vi "Determine Where to Add.vi"(8 "error in (no error)":errorcluster, 11 "QControlWizard in":refnum<class "QControl Creation Wizard.lvclass">) -> (0 "error out":errorcluster, 3 "QControlWizard (dup)":refnum<class "QControl Creation Wizard.lvclass">)   [LabVIEW 2015, in "QControl Creation Wizard.lvclass"]
doc: "<b> </b> <b> </b>\n©2016 Q Software Innovations, LLC (QSI)\nwritten by Quentin Alldredge\nproduced in LabVIEW 2015\n\nsupport@qsoftwareinnovations.com\nwww.qsoftwareinnovations.com\n\nAll rights reserved.\n\nRedistribution and use in source and binary forms, with or without modification, are permitted provided that the following conditions are met:\n\n * Redistributions of source code must retain the above copyright notice, this list of conditions and the following disclaimer.\n * Redistributions in binary form must reproduce the above copyright notice, this list of conditions and the following disclaimer in the documentation and/or other materials provided with the distribution.\n * Neither the name of Q Software Innovations, LLC. nor the names of its contributors may be used to endorse or promote products derived from this software without specific prior written permission.\n\nTHIS SOFTWARE IS PROVIDED BY THE COPYRIGHT HOLDERS AND CONTRIBUTORS \"AS IS\" AND ANY EXPRESS OR IMPLIED WARRANTIES, INCLUDING, BUT NOT LIMITED TO, THE IMPLIED WARRANTIES OF MERCHANTABILITY AND FITNESS FOR A PARTICULAR PURPOSE ARE DISCLAIMED. IN NO EVENT SHALL THE COPYRIGHT OWNER OR CONTRIBUTORS BE LIABLE FOR ANY DIRECT, INDIRECT, INCIDENTAL, SPECIAL, EXEMPLARY, OR CONSEQUENTIAL DAMAGES (INCLUDING, BUT NOT LIMITED TO, PROCUREMENT OF SUBSTITUTE GOODS OR SERVICES; LOSS OF USE, DATA, OR PROFITS; OR BUSINESS INTERRUPTION) HOWEVER CAUSED AND ON ANY THEORY OF LIABILITY, WHETHER IN CONTRACT, STRICT LIABILITY, OR TORT (INCLUDING NEGLIGENCE OR OTHERWISE) ARISING IN ANY WAY OUT OF THE USE OF THIS SOFTWARE, EVEN IF ADVISED OF THE POSSIBILITY OF SUCH DAMAGE."
uses:
  QControl Creation Wizard.lvclass
  QControl Creation Wizard.lvclass/QControl Creation Wizard.ctl
  New QControl Info/New QControl Info.lvclass/New QControl Info.ctl
  New QControl Info/Write Add to Location.vi
  New QControl Info/Write ProjectItem Ref.vi
  New QControl Info/Write Target Ref.vi
  New QControl Info/Read App Refnum.vi
  New QControl Info/New QControl Info.lvclass
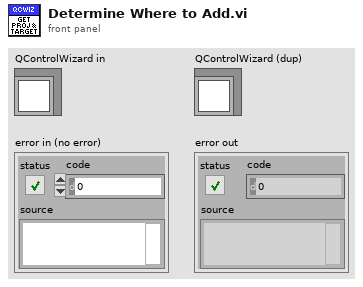
[diagram p1: front panel]
types:
  T1 = enum16{"Don't Add", "To Target", "To Project Item"}
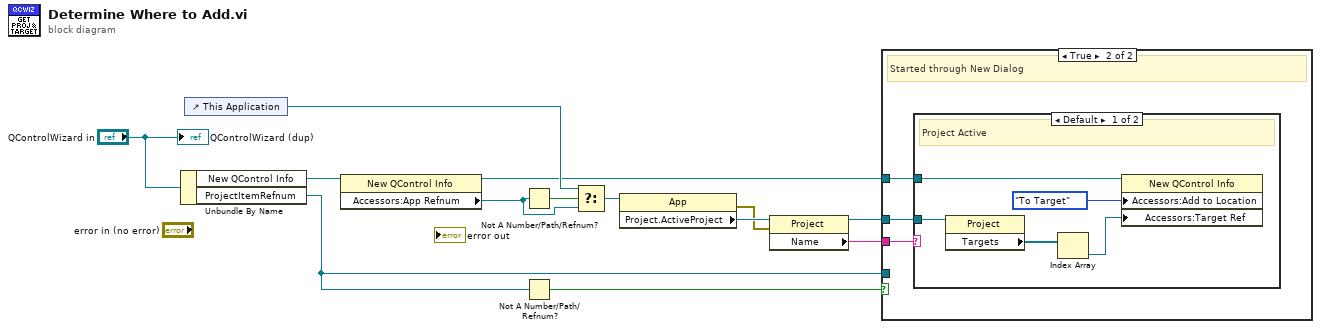
[diagram p0: block diagram]
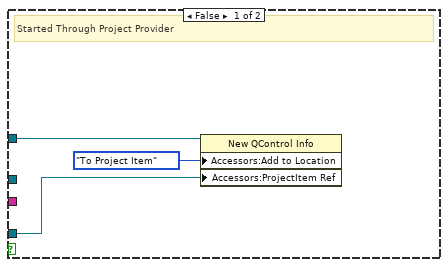
[diagram p2: hidden frame]
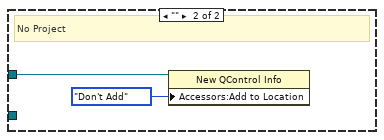
[diagram p3: hidden frame]
diagram:
  n1 = Unbundle By Name("QControlWizard in") -> ("New QControl Info"=w4:refnum<data-value>, "ProjectItemRefnum"=w5:refnum<vi>)
  n2 = control-ref of="This Application"() -> (w9:refnum<vi>)
  n3 = property class="New QControl Info"(reference=w4) -> (reference out=w2:refnum<data-value>, "Accessors:App Refnum"=w1:refnum<vi>)  [unwired: 1 in, 1 out]
  n4 = Not A Number/Path/Refnum?(number/path/refnum=w1) -> (NaN/Path/Refnum?=w11:bool)
  n5 = Not A Number/Path/Refnum?(number/path/refnum=w5) -> (NaN/Path/Refnum?=w7:bool)
  n6 = Select(t=w9, s=w11, f=w1) -> (s? t:f=w10:refnum<vi>)
  n7 = property class="App"(reference=w10) -> (error out=w12:errorcluster, "Project.ActiveProject"=w13:refnum<vi>)  [unwired: 1 in, 1 out]
  n8 = property class="Project"(reference=w13, error in=w12) -> (reference out=w6:refnum<vi>, "Name"=w8:string)  [unwired: 1 out]
  n9 = case shown="True" w7 {
    tunnel: w8 -> [_ w19]
    tunnel: w6 -> [_ w18]
    tunnel: w5 -> [w15 _]
    tunnel: w2 -> [w14 w17]
    frame False {
      # "Started Through Project Provider"
      n10 = property class="New QControl Info"(reference=w14, "Accessors:Add to Location"=T1."To Project Item" ("Add to Location"), "Accessors:ProjectItem Ref"=w15) -> ()  [unwired: 1 in, 2 out]
    }
    frame True {
      # "Started through New Dialog"
      n11 = case shown="Default" w19 {
        tunnel: w18 -> [w23 _]
        tunnel: w17 -> [w22 w26]
        frame Default {
          # "Project Active"
          n12 = property class="Project"(reference=w23) -> ("Targets"=w24:refnum<vi>[])  [unwired: 1 in, 2 out]
          n13 = Index Array(array=w24) -> (element=w21:refnum<vi>)  [unwired: 1 in]
          n14 = property class="New QControl Info"(reference=w22, "Accessors:Add to Location"=T1."To Target" ("Add to Location"), "Accessors:Target Ref"=w21) -> ()  [unwired: 1 in, 2 out]
        }
        frame "" {
          # "No Project"
          n15 = property class="New QControl Info"(reference=w26, "Accessors:Add to Location"=T1."Don't Add" ("Add to Location")) -> ()  [unwired: 1 in, 2 out]
        }
      }
    }
  }
  "QControlWizard (dup)" <- "QControlWizard in"
